vi "ExecuteAction.vi"(8 "ErrorIn":errorcluster, 10 "ButtonDefinition":T1, 11 "VerticalButtonBarIn":refnum<class "VerticalButtonBar.lvclass">) -> (0 "ErrorOut":errorcluster, 3 "VerticalButtonBarOut":refnum<class "VerticalButtonBar.lvclass">)   [LabVIEW 2021, in "VerticalButtonBar.lvclass"]
uses:
  VerticalButtonBar.lvclass
  ButtonCollection/ButtonDefinition.ctl
  Interface_TAF_ITAFGUIActions/ITAFGUIActions/ITAFGUIActions.lvclass
  e2e359f8-865c-46d2-be85-a7a6c724827c.vi
  81b4402e-c7ae-47ab-bf16-de1b2dba09db.vi
  <vilib>/TriekselSoft/TracerLibrary/TracerLibrary/Tracer/protected/SendMessage.vi
  <vilib>/TriekselSoft/TracerLibrary/TracerLibrary/Tracer/protected/Timestamp.vi
  e2e359f8-865c-46d2-be85-a7a6c724827c.vi/f75db090-0877-4668-94fb-75c2140b1617.vi
  81b4402e-c7ae-47ab-bf16-de1b2dba09db.vi/f75db090-0877-4668-94fb-75c2140b1617.vi
  <vilib>/TriekselSoft/TracerLibrary/TracerLibrary/Tracer/Tracer_Level-Info.vi
  <vilib>/JDP Science/JSONtext/Variant to JSON Text.vi
  <vilib>/TriekselSoft/TracerLibrary/TracerLibrary/Tracer/protected/Tracer_ClassAttributes.vi
  <vilib>/JDP Science/JSONtext/LVClass Serializer/JSONtext LVClass Serializer.lvclass
  Interface_UserInterface_IDockGUI/IDockGUI/IDockGUI.lvclass
  VerticalButtonBar.lvclass/VerticalButtonBar.ctl
  Library_TAF_ApplicationFramework/Application/Application.lvclass
  ButtonCollection/ButtonCollection.lvclass
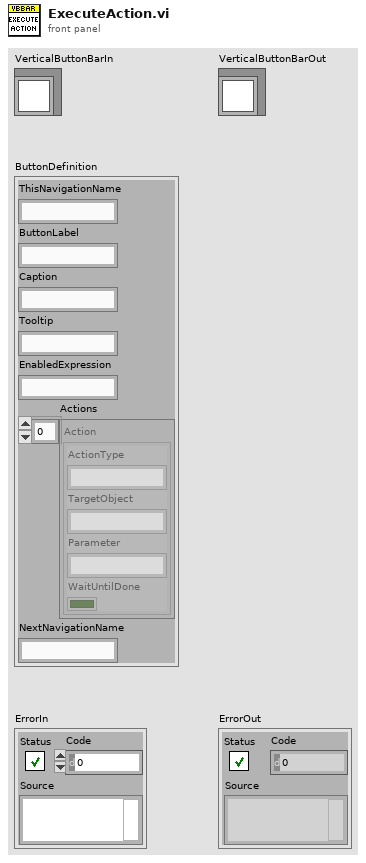
[diagram p1: front panel]
types:
  T1 = typedef "ButtonCollection.lvclass/ButtonDefinition.ctl" = cluster{"ThisNavigationName":string, "ButtonLabel":string, "Caption":string, "Tooltip":string, "EnabledExpression":string, "Actions":cluster{"ActionType":string, "TargetObject":string, "Parameter":string, "WaitUntilDone":bool}[], "NextNavigationName":string}
  T2 = typedef "VerticalButtonBar.lvclass/ObjectAttributes.ctl" = cluster{"Interfaces":cluster{"IDockGUI":refnum<class "IDockGUI.lvclass">, "Authorizer":refnum<class "IAuthorization.lvclass">}, "Locals":cluster{"ButtonBar":refnum<class "ButtonCollection.lvclass">, "BaseConfigurationPath":path, "Labels":cluster{"Label":string, "Value":string}[]}, "Persistent":cluster{"ButtonDefinitionFile":string}}
  T3 = cluster{"ActionType":string, "TargetObject":string, "Parameter":string, "WaitUntilDone":bool}[]
  T4 = cluster{"ButtonLabel":string, "Caption":string, "Action":cluster{"ActionType":string, "TargetObject":string, "Parameter":string, "WaitUntilDone":bool}}
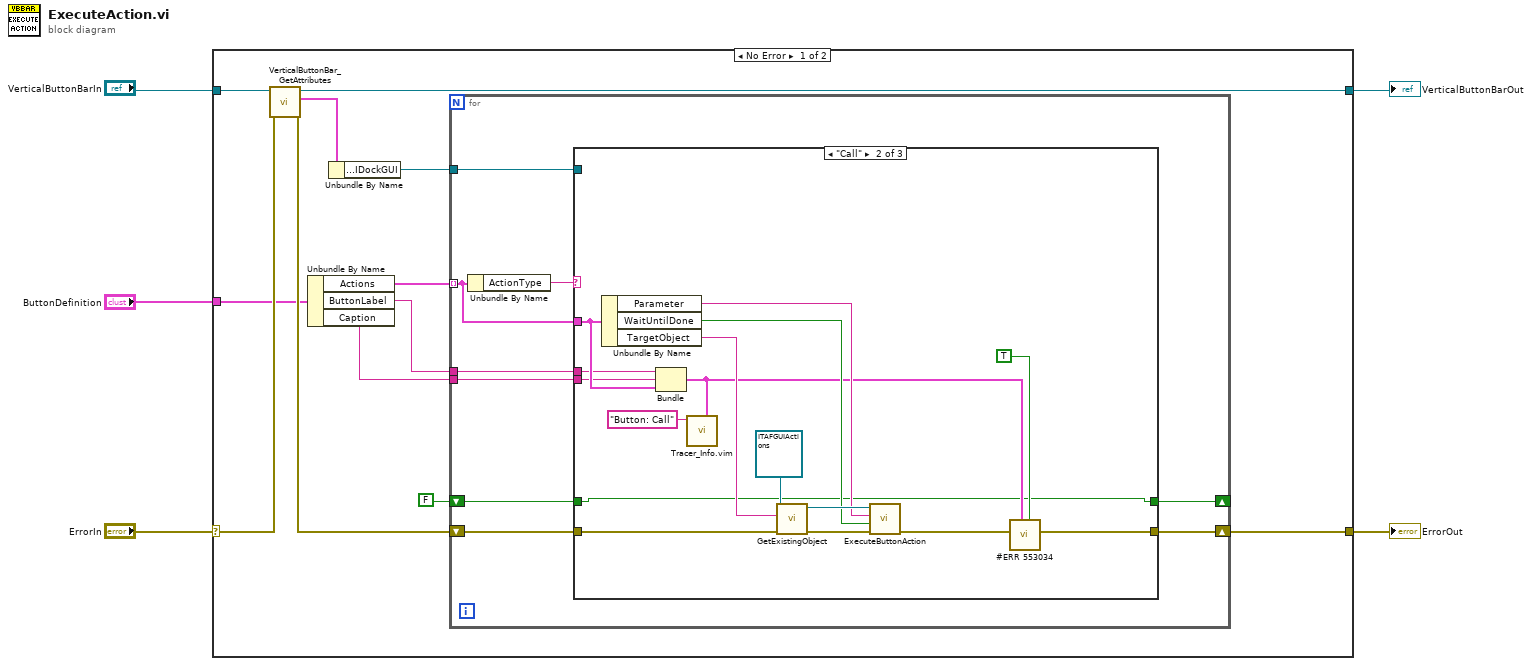
[diagram p0: block diagram]
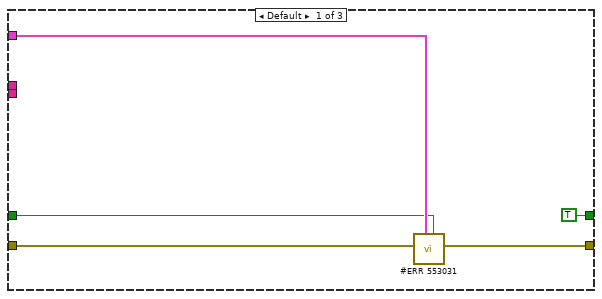
[diagram p2: hidden frame]
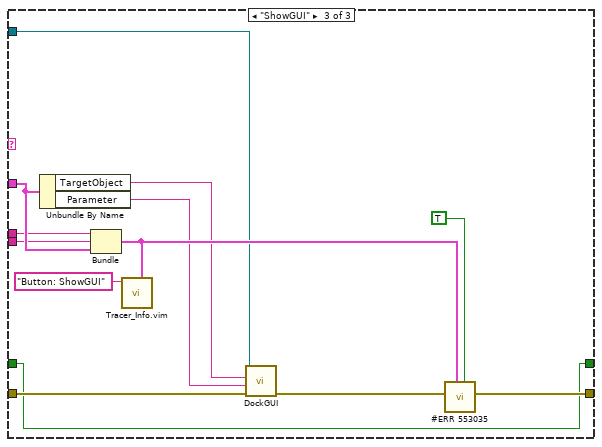
[diagram p3: hidden frame]
diagram:
  n1 = case shown="No Error" "ErrorIn" {
    selector: "ErrorIn" -> [w16 w62]
    tunnel: [w17 w62] -> w4
    tunnel: "ButtonDefinition" -> [w14 _]
    tunnel: "VerticalButtonBarIn" -> [w10 w61]
    tunnel: [w9 w61] -> w1
    frame No Error {
      n2 = call "VerticalButtonBar_GetAttributes.vi"("ErrorIn"=w16, "ReferenceIn"=w10) -> ("ErrorOut"=w15:errorcluster, "Data"=w8:T2, "ReferenceOut"=w9:refnum<class "VerticalButtonBar.lvclass">)  [unwired: 6 in, 1 out]
      n3 = Unbundle By Name(w14) -> ("Actions"=w13:T3, "ButtonLabel"=w11:string, "Caption"=w12:string)
      n4 = Unbundle By Name(w8) -> ("Interfaces.IDockGUI"=w7:refnum<class "IDockGUI.lvclass">)
      n5 = for {
        tunnel: w13 -> [w23] mode=indexing
        shift-right: [w25] -> w17
        shift-left: w15 -> [w26]
        tunnel: w12 -> [w22]
        tunnel: w11 -> [w21]
        tunnel: w7 -> [w20]
        shift-right: [w18] -> _
        shift-left: FALSE -> [w19]
        n6 = Unbundle By Name(w23) -> ("ActionType"=w24:string)
        n7 = case shown="\"Call\"" w24 {
          tunnel: [w31 w44 w60] -> w25
          tunnel: w26 -> [w30 w47 w59]
          tunnel: w23 -> [w29 w37 w56]
          tunnel: w22 -> [_ w36 w55]
          tunnel: w21 -> [_ w35 w54]
          tunnel: w20 -> [_ _ w49]
          tunnel: w19 -> [w28 w32 w48]
          tunnel: [TRUE w32 w48] -> w18
          frame Default {
            n8 = call "#ERR 553031"("MergeErrors"=w28, "Data"=w29, "error in (no error)"=w30) -> ("error out"=w31:errorcluster)  [unwired: 8 in]
          }
          frame "Call" {
            n9 = Unbundle By Name(w37) -> ("Parameter"=w39:string, "WaitUntilDone"=w40:bool, "TargetObject"=w43:string)
            n10 = Bundle("ButtonLabel"=w35, "Caption"=w36, "Action"=w37) -> (w34:T4)  [unwired: 1 in]
            n11 = call "Tracer_Info.vim"("Data"=w34, "Info Text"="Button: Call" ("InfoText")) -> ()  [unwired: 9 in, 1 out]
            n12 = call "GetExistingObject.vi"("ErrorIn"=w47, "ObjectName"=w43, "Type"=refnum<class "ITAFGUIActions.lvclass"> refnum ("ButtonAction")) -> ("ErrorOut"=w46:errorcluster, "ObjectOut"=w41:refnum<class "ITAFGUIActions.lvclass">)  [unwired: 7 in]
            n13 = call-dynamic "ExecuteButtonAction.vi"("ErrorIn"=w46, "WaitForReply"=w40, "Command"=w39, "ObjectIn"=w41) -> ("ErrorOut"=w45:errorcluster)  [unwired: 6 in, 1 out]
            n14 = call "#ERR 553034"("MergeErrors"=TRUE, "Data"=w34, "error in (no error)"=w45) -> ("error out"=w44:errorcluster)  [unwired: 8 in]
          }
          frame "ShowGUI" {
            n15 = Unbundle By Name(w56) -> ("TargetObject"=w51:string, "Parameter"=w50:string)
            n16 = Bundle("ButtonLabel"=w54, "Caption"=w55, "Action"=w56) -> (w53:T4)  [unwired: 1 in]
            n17 = call "Tracer_Info.vim"("Data"=w53, "Info Text"="Button: ShowGUI" ("InfoText")) -> ()  [unwired: 9 in, 1 out]
            n18 = call-dynamic "DockGUI.vi"("ErrorIn"=w59, "SubPanelName"=w50, "ObjectName"=w51, "ObjectIn"=w49) -> ("ErrorOut"=w58:errorcluster)  [unwired: 6 in, 1 out]
            n19 = call "#ERR 553035"("MergeErrors"=TRUE, "Data"=w53, "error in (no error)"=w58) -> ("error out"=w60:errorcluster)  [unwired: 8 in]
          }
        }
      }
    }
    frame Error {
    }
  }
  "ErrorOut" <- w4
  "VerticalButtonBarOut" <- w1
